vi "test no ppl.vi"(8 "error in (no error)":errorcluster, 11 "TestCase in":refnum<class "Configure RunTime Path Tests.lvclass">) -> (0 "error out":errorcluster, 3 "TestCase out":refnum<class "Configure RunTime Path Tests.lvclass">)   [LabVIEW 2017, in "Configure RunTime Path Tests.lvclass"]
uses:
  Configure RunTime Path Tests.lvclass
  <vilib>/addons/_JKI Toolkits/VI Tester/TestCase.llb/TestCase.lvclass
  TSC File IO.lvlib
  C:/Program Files (x86)/National Instruments/LabVIEW 2017/vi.lib/addons/_JKI Toolkits/VI Tester/TestCase.llb/TestCase.lvclass
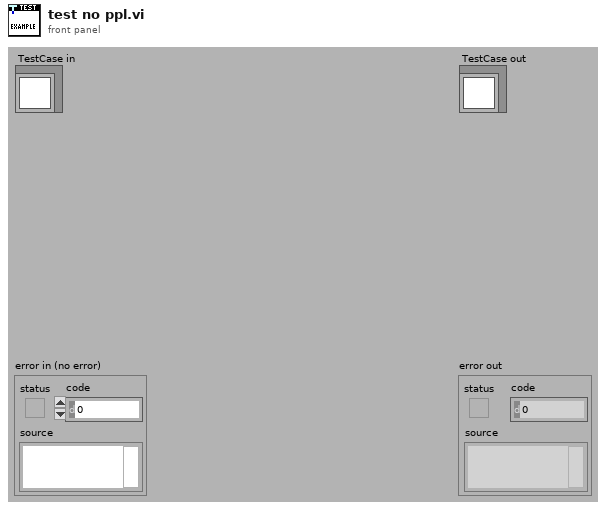
[diagram p1: front panel]
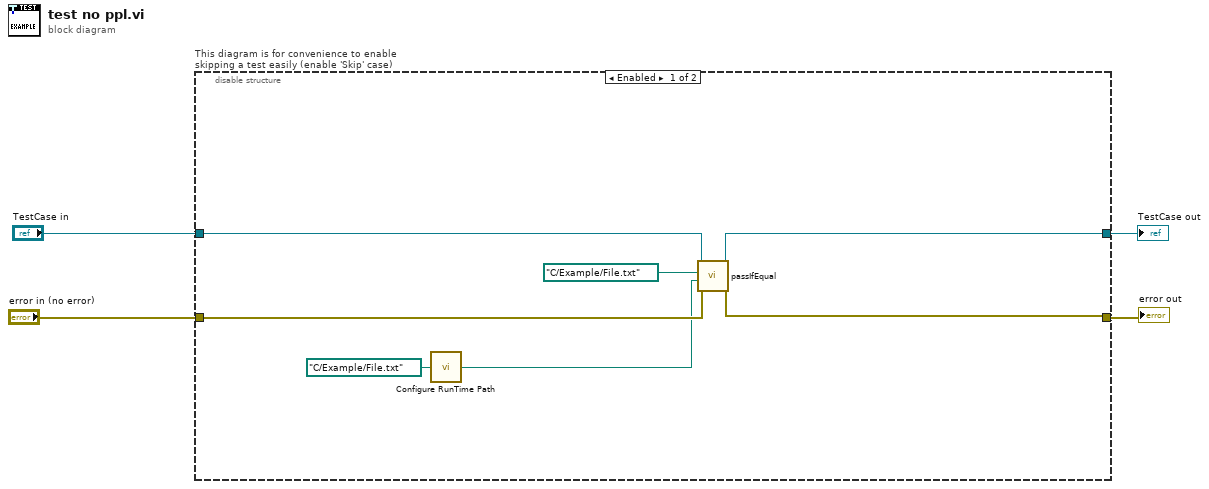
[diagram p0: block diagram]
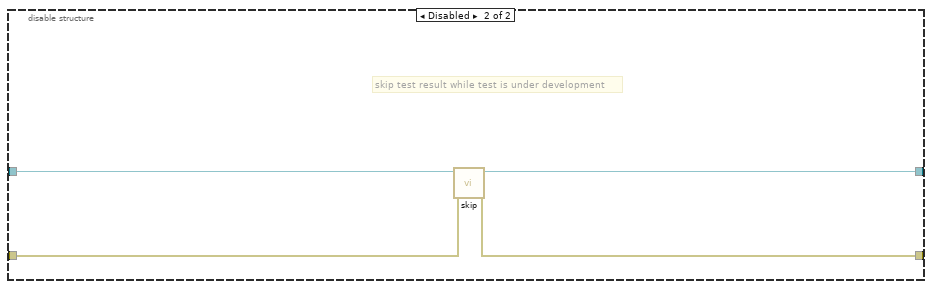
[diagram p2: hidden frame]
diagram:
  n1 = disable-structure "This diagram is for convenience to enable skipping a test easily (enable 'Skip' case)" shown="Enabled" {
    disable-tunnel: "TestCase in" -> [w11 w15]
    disable-tunnel: [w10 w13] -> w1
    disable-tunnel: [w9 w14] -> w3
    disable-tunnel: "error in (no error)" -> [w8 w12]
    frame Enabled {
      n2 = call "Configure RunTime Path.vi"("Input Path"=path "C:/Example/File.txt") -> ("Updated Path"=w6:path)
      n3 = call-dynamic "passIfEqual.vi"("error in (no error)"=w8, "y"=w6, "x"=path "C:/Example/File.txt", "TestCase in"=w11) -> ("error out"=w9:errorcluster, "TestCase out"=w10:refnum<class "Configure RunTime Path Tests.lvclass">)  [unwired: 6 in]
    }
    frame Disabled {
      # "skip test result while test is under development"
      n4 = call <vilib>:"skip.vi"("error in (no error)"=w12, "TestCase in"=w15) -> ("error out"=w14:errorcluster, "TestCase out"=w13:refnum<class "Configure RunTime Path Tests.lvclass">)  [unwired: 8 in]
    }
  }
  "error out" <- w3
  "TestCase out" <- w1
